vi "Correl_calc.vi"() -> ()   [LabVIEW 2013]
uses:
  <vilib>/Utility/file.llb/Write To Spreadsheet File (DBL).vi
  <vilib>/Utility/file.llb/Read From Spreadsheet File (I64).vi
  <vilib>/Utility/file.llb/Read From Spreadsheet File (DBL).vi
  <vilib>/gmath/NI_Gmath.lvlib
panel:
  out "size(s)":i32
  in  "피험자_이름":string
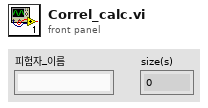
[diagram p1: front panel]
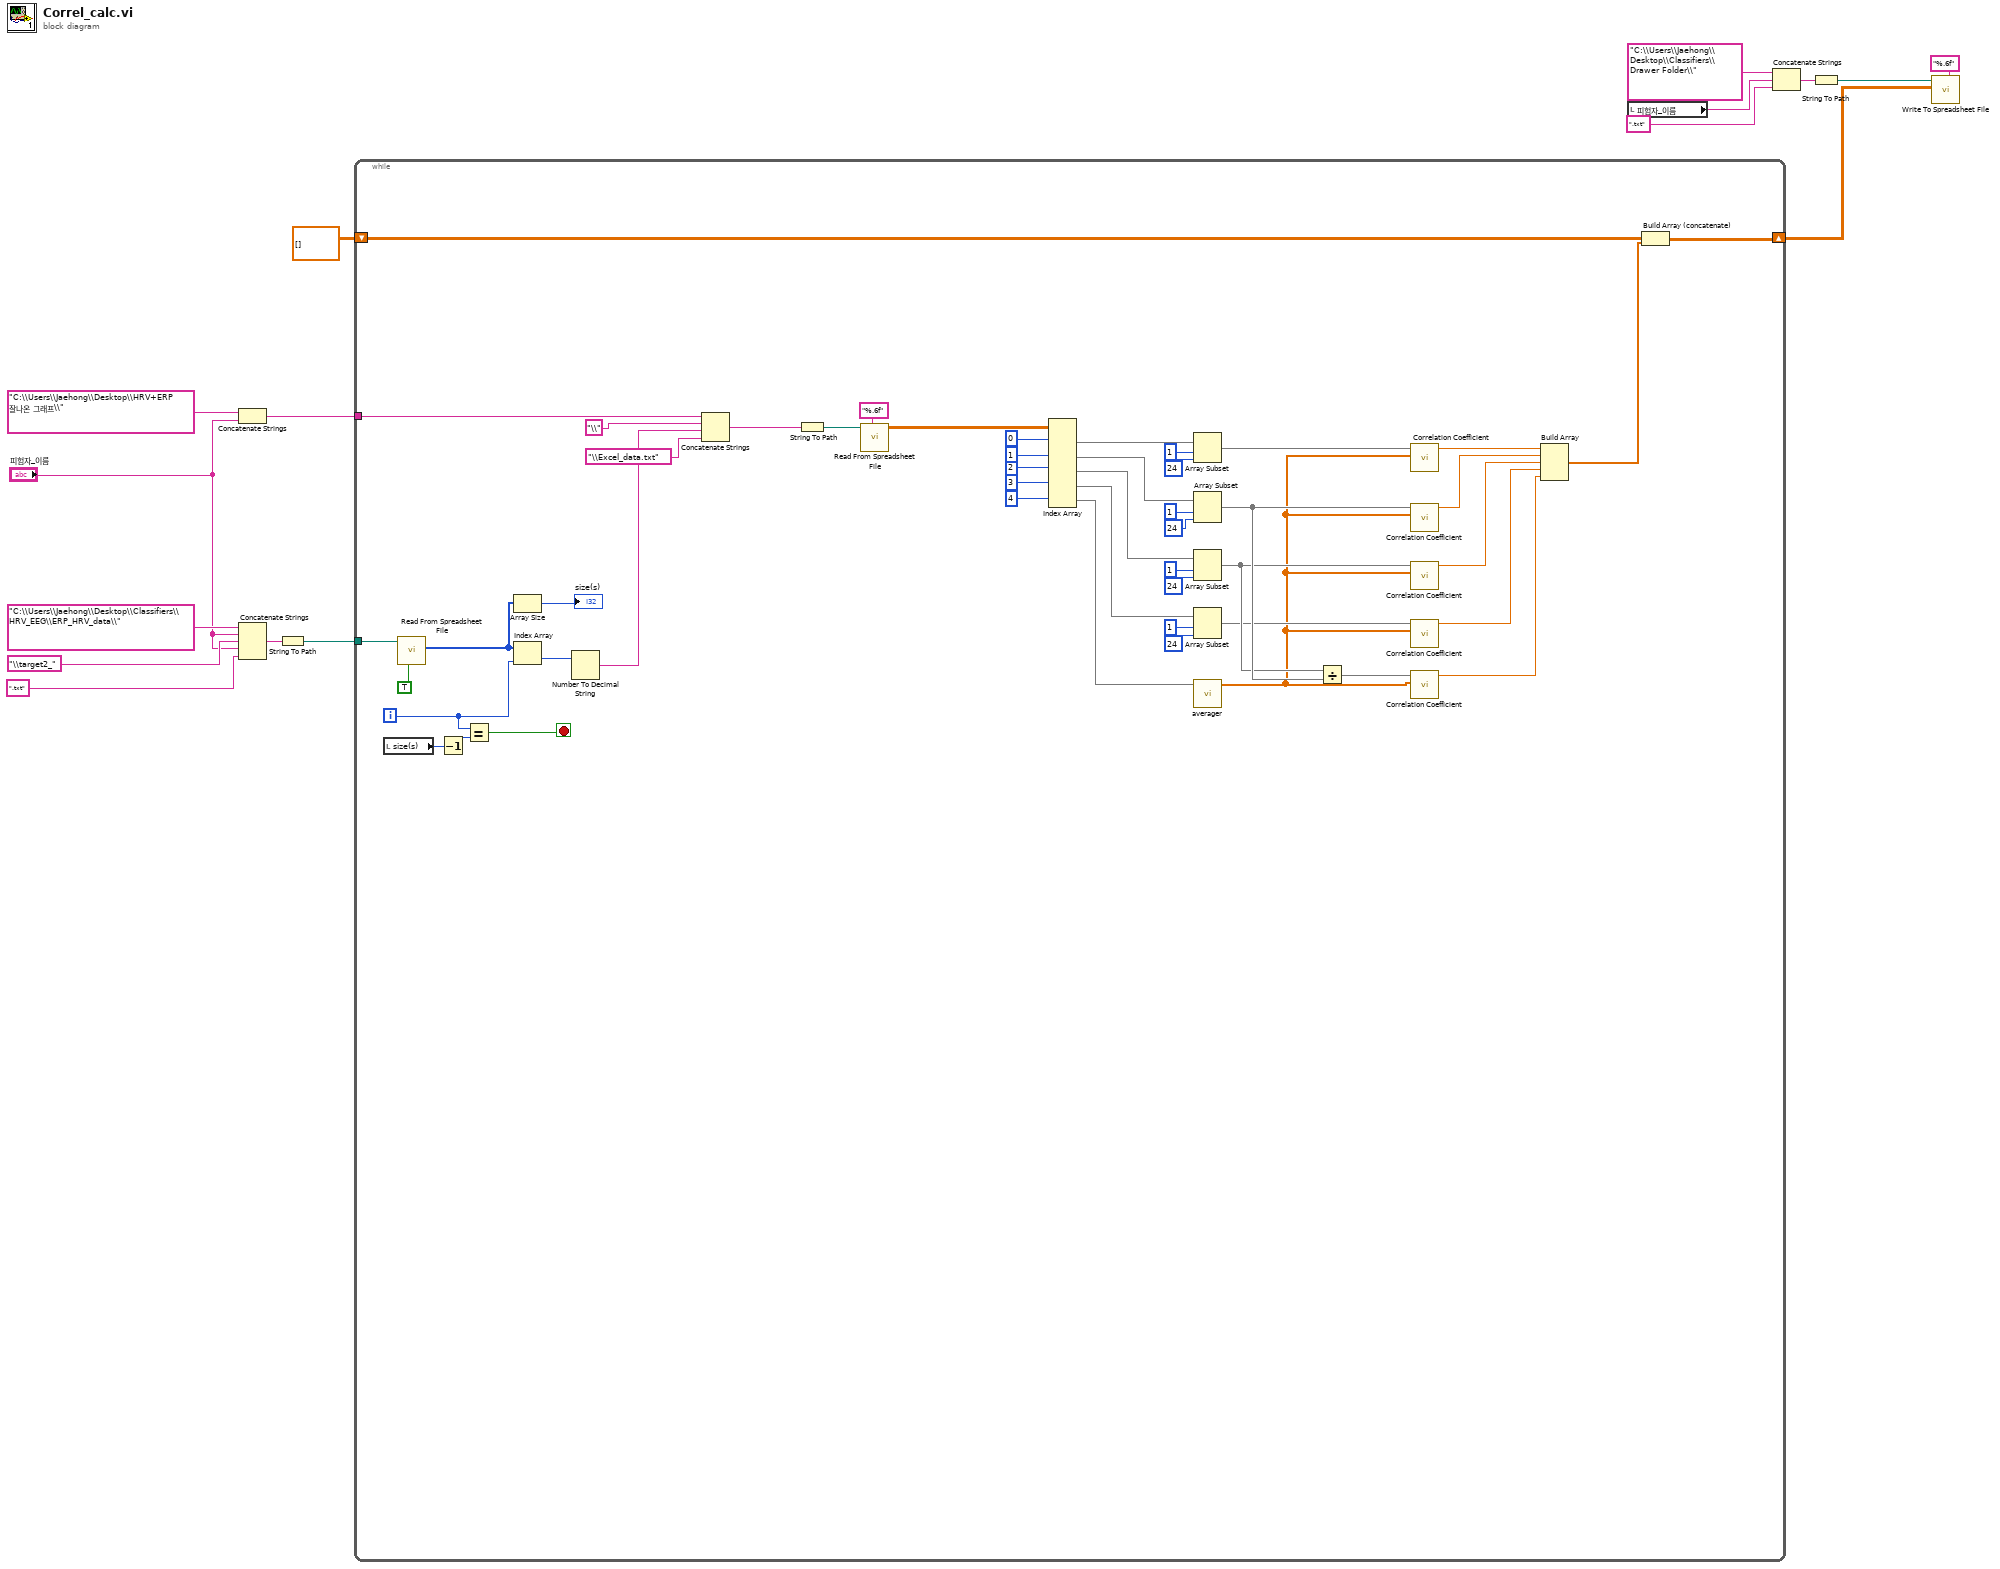
[diagram p0: block diagram]
diagram:
  n1 = Concatenate Strings("C:\\Users\\Jaehong\\Desktop\\HRV+ERP 잘나온 그래프\\", "피험자_이름") -> (w15:string)
  n2 = Concatenate Strings("C:\\Users\\Jaehong\\Desktop\\Classifiers\\HRV_EEG\\ERP_HRV_data\\", "피험자_이름", "\\target2_", "피험자_이름", ".txt") -> (w10:string)
  n3 = String To Path(string=w10) -> (path=w9:path)
  n4 = while {
    tunnel: w15 -> [w63]
    tunnel: w9 -> [w65]
    shift-right: [w19] -> w2
    shift-left: dbl[][] [] -> [w18]
    i -> [w23]
    stop <- w21 stop-if-true
    n5 = local read "size(s)"() -> (w22:i32)
    n6 = call-poly <vilib>:"Read From Spreadsheet File.vi"("transpose (no:F)"=TRUE, "file path (dialog if empty)"=w65) -> ("first row"=w36:i64[])  [unwired: 5 in, 4 out]
    n7 = Decrement(x=w22) -> (x-1=w17:i32)
    n8 = Equal?(x=w23, y=w17) -> (x = y?=w21:bool)
    n9 = Array Size(array=w36) -> (size(s)=→"size(s)":i32)
    n10 = Index Array(array=w36, index=w23) -> (element=w61:i64)
    n11 = Number To Decimal String(number=w61) -> (decimal integer string=w60:string)  [unwired: 1 in]
    n12 = Concatenate Strings(w63, "\\", w60, "\\Excel_data.txt") -> (w58:string)
    n13 = String To Path(string=w58) -> (path=w57:path)
    n14 = call-poly <vilib>:"Read From Spreadsheet File.vi"("format (%.3f)"="%.6f", "file path (dialog if empty)"=w57) -> ("all rows"=w55:dbl[][])  [unwired: 5 in, 4 out]
    n15 = Index Array(array=w55, index (row) #1=0 ("index (row)"), index (row) #2=1 ("index (row)"), index (row) #3=2 ("index (row)"), index (row) #4=3 ("index (row)"), index (row) #5=4 ("index (row)")) -> (element #1=w49:dbl[], element #2=w40:dbl[], element #3=w39:dbl[], element #4=w38:dbl[], element #5=w37:dbl[])  [unwired: 5 in]
    n16 = Array Subset(array=w49, index=1, length=24) -> (w34:dbl[])
    n17 = Array Subset(array=w40, index=1, length=24) -> (w33:dbl[])
    n18 = Array Subset(array=w39, index=1, length=24) -> (w32:dbl[])
    n19 = Array Subset(array=w38, index=1, length=24) -> (w31:dbl[])
    n20 = call "averager.vi"("input"=w37) -> ("output"=w29:dbl[])  [unwired: 10 in]
    n21 = Divide(x=w32, y=w33) -> (x/y=w30:dbl[])
    n22 = call <vilib>:"Correlation Coefficient.vi"("Y"=w29, "X"=w34) -> ("correlation coefficient r"=w28:dbl)  [unwired: 8 in, 1 out]
    n23 = call <vilib>:"Correlation Coefficient.vi"("Y"=w29, "X"=w33) -> ("correlation coefficient r"=w27:dbl)  [unwired: 8 in, 1 out]
    n24 = call <vilib>:"Correlation Coefficient.vi"("Y"=w29, "X"=w32) -> ("correlation coefficient r"=w26:dbl)  [unwired: 8 in, 1 out]
    n25 = call <vilib>:"Correlation Coefficient.vi"("Y"=w29, "X"=w31) -> ("correlation coefficient r"=w25:dbl)  [unwired: 8 in, 1 out]
    n26 = call <vilib>:"Correlation Coefficient.vi"("Y"=w29, "X"=w30) -> ("correlation coefficient r"=w24:dbl)  [unwired: 8 in, 1 out]
    n27 = Build Array(w28, w27, w26, w25, w24) -> (w20:dbl[])
    n28 = Build Array (concatenate)(w18, w20) -> (w19:dbl[][])
  }
  n29 = local read "피험자_이름"() -> (w6:string)
  n30 = Concatenate Strings("C:\\Users\\Jaehong\\Desktop\\Classifiers\\Drawer Folder\\", w6, ".txt") -> (w4:string)
  n31 = String To Path(string=w4) -> (path=w3:path)
  n32 = call-poly <vilib>:"Write To Spreadsheet File.vi"("format (%.3f)"="%.6f", "2D data"=w2, "file path (dialog if empty)"=w3) -> ()  [unwired: 5 in, 1 out]
